vi "Turn To Angle.vi"(10 "Current Angle":dbl, 11 "Target Angle":dbl) -> (0 "Finished":bool)   [LabVIEW 2015]
uses:
  <vilib>/Rock Robotics/WPI/Utilities/WPI_GetSetVariantRefNum.vi
  <vilib>/addons/control/pid/pid.llb/PID (DBL).vi
  <vilib>/Rock Robotics/WPI/RobotDrive/WPI_RobotDriveArcadeDrive_Standard(NoSaturation).vi
  <vilib>/addons/control/pid/NI_PID_pid.lvlib
panel:
  in  "PID gains":T1={"proportional gain (Kc)"=1.0, "integral time (Ti, min)"=0.0, "derivative time (Td, min)"=0.0} {"derivative time (Td, min)" format="%.3f"; "integral time (Ti, min)" format="%.3f"; "proportional gain (Kc)" format="%.3f"}
  in  "Min":dbl=0.5
  in  "Max":dbl=0.75
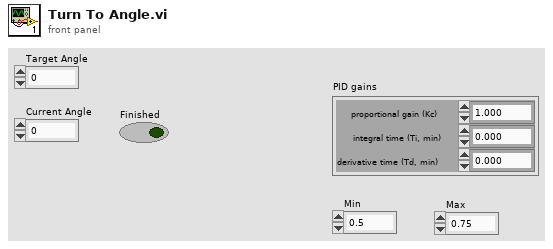
[diagram p1: front panel]
types:
  T1 = cluster{"proportional gain (Kc)":dbl, "integral time (Ti, min)":dbl, "derivative time (Td, min)":dbl}
  T2 = typedef "WPI_RobotDriveDevRef.ctl" = cluster{"DevStatus":errorcluster, "Motors[]":T3[], "Square Inputs":bool, "Max Output":dbl}
  T3 = typedef "WPI_MotorControlDeviceRef.ctl" = cluster{"DeviceStatus":errorcluster, "Type":T4, "PWM":cluster{"PWM Channel":T5, "DeadBand":T6}, "CAN":cluster{"Device Number":u8, "Control Mode":T7, "Semaphore":T8, "Max Vout":dbl, "TalonSRX Control Mode":T9}, "Invert":bool}
  T4 = typedef "WPI_MotorControlType.ctl" = enum16{"PWM", "CAN", "CANTalonSRX"}
  T5 = typedef "FPGA_DIOPWMChannel.ctl" = enum8{"PWM 0", "PWM 1", "PWM 2", "PWM 3", "PWM 4", "PWM 5", "PWM 6", "PWM 7", "PWM 8", "PWM 9", "PWM MXP 0", "PWM MXP 1", "PWM MXP 2", "PWM MXP 3", "PWM MXP 4", "PWM MXP 5", "PWM MXP 6", "PWM MXP 7", "PWM MXP 8", "PWM MXP 9", "Invalid"}
  T6 = typedef "WPI_PWMDeadband.ctl" = cluster{"Name":string, "maxPositivePwm":i32, "minPositivePwm":i32, "centerPwm":i32, "maxNegativePwm":i32, "minNegativePwm":i32, "angularRange":u16}
  T7 = typedef "WPI_CANJaguar_ControlMode.ctl" = enum8{"Percent VBus", "Current", "Speed", "Position", "Voltage"}
  T8 = typedef "Semaphore RefNum" = refnum<k1>
  T9 = typedef "WPI_CANTalonSRX_APIControlMode.ctl" = enum8{"Percent VBus", "Speed", "Position", "Slave", "Unchanged / Invalid", "Voltage Compensation", "Current", "Motion Profile"}
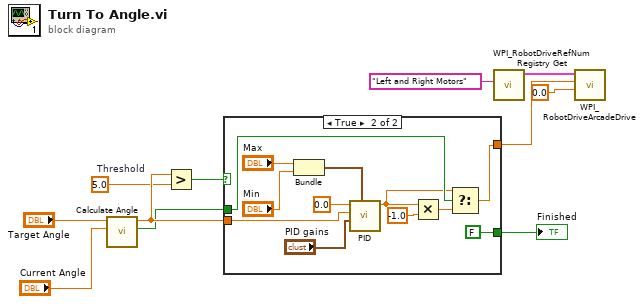
[diagram p0: block diagram]
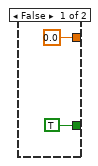
[diagram p2: hidden frame]
diagram:
  w3 = 5.0  # Threshold
  n1 = call "Calculate Angle.vi"("Current Angle"="Current Angle", "Target Angle"="Target Angle") -> ("Clockwise"=w6:bool, "Delta Angle"=w7:dbl)  [unwired: 8 in]
  n2 = Greater?(x=w7, y=w3) -> (0:w2:bool)
  n3 = case shown="True" w2 {
    tunnel: [0.0 ("Left axis value") w24] -> w8
    tunnel: w6 -> [_ w23]
    tunnel: [TRUE ("Rotate Enabled") FALSE ("Rotate Enabled")] -> w1
    tunnel: w7 -> [_ w19]
    frame False {
    }
    frame True {
      n4 = Bundle("Max"="Max", "Min"="Min") -> (w15:cluster{"Max":dbl, "Min":dbl})  [unwired: 1 in]
      n5 = call-poly <vilib>:"PID.vi"("output range"=w15, "PID gains"="PID gains", "process variable"=w19, "setpoint"=0.0) -> ("output"=w20:dbl)  [unwired: 6 in, 1 out]
      n6 = Multiply(x=w20, y=-1.0) -> (x*y=w22:dbl)
      n7 = Select(t=w20, s=w23, f=w22) -> (s? t:f=w24:dbl)
    }
  }
  "Finished" <- w1
  n8 = call <vilib>:"WPI_RobotDriveRefNum Registry Get.vi"("refnum name"="Left and Right Motors") -> ("RobotDriveDevRef"=w11:T2)  [unwired: 1 in, 9 out]
  n9 = call-poly <vilib>:"WPI_RobotDriveArcadeDrive.vi"("Y axis value"=0.0, "X axis value"=w8, "RobotDriveDevRef"=w11) -> ()  [unwired: 6 in, 3 out]
